vi "Initialize MeasurementLink Session.vi"(7 "remote connection options":T2, 8 "error in":errorcluster, 9 "initialize and close session behavior":T1, 10 "session initialization parameters":T3, 11 "session factory in":refnum<class "Keysight_34401A-DMM.lvclass">) -> (0 "error out":errorcluster, 2 "session out":variant, 3 "session factory out":refnum<class "Keysight_34401A-DMM.lvclass">)   [LabVIEW 2020, in "Keysight_34401A-DMM.lvclass"]
doc: "Creates a new session using the provided <b>session initialization parameters</b>. If the session represents a remote session, <b>initialize and close session behavior</b> determines whether creating the local session creates a new session on the server or attaches to an existing session on the server."
uses:
  Keysight_34401A-DMM.lvclass
  <vilib>/MeasurementLink/MeasurementLink Instrument/ISession Factory/Session Initialization Parameters.ctl
  <vilib>/MeasurementLink/MeasurementLink Instrument/ISession Factory/Remote Connection Options.ctl
  <vilib>/MeasurementLink/MeasurementLink Instrument/ISession Factory/Initialize and Close Session Behavior.ctl
  Keysight_34401A-DMM.lvclass/Keysight_34401A-DMM.ctl
  <vilib>/MeasurementLink/MeasurementLink Instrument/ISession Factory/ISession Factory.lvclass
  <instrlib>/Agilent 34401/Public/Initialize.vi
  <instrlib>/Agilent 34401/Agilent 34401.lvlib
  SubVI/Get VISA gRPC Open Close Behavior.vi
  <vilib>/NI-VISA/VISA Open for gRPC Session.vi
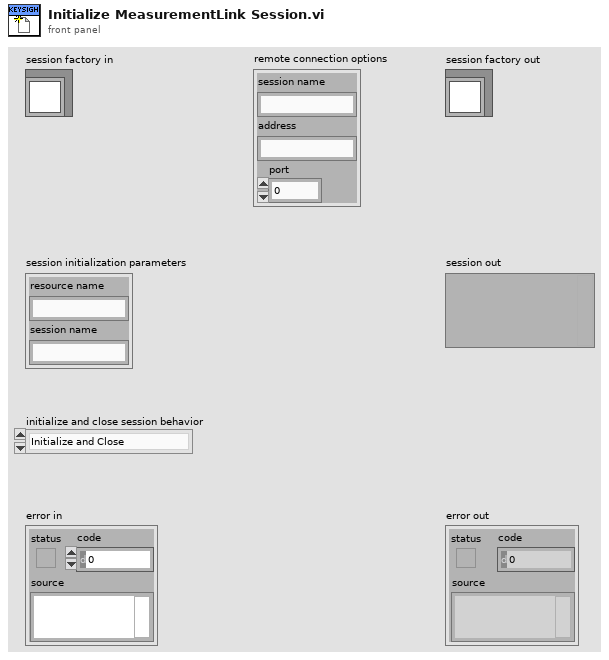
[diagram p1: front panel]
types:
  T1 = typedef "MeasurementLink Instrument.lvlib/ISession Factory.lvclass/Initialize and Close Session Behavior.ctl" = enum16{"Initialize and Close", "Attach and Detach", "Initialize and Detach", "Attach and Close"}
  T2 = typedef "MeasurementLink Instrument.lvlib/ISession Factory.lvclass/Remote Connection Options.ctl" = cluster{"session name":string, "address":string, "port":u32}
  T3 = typedef "MeasurementLink Instrument.lvlib/ISession Factory.lvclass/Session Initialization Parameters.ctl" = cluster{"resource name":string, "session name":string}
  T4 = typedef "VISA gRPC Open Close Behavior.ctl" = enum16{"Auto", "Initialize and Close", "Attach and Detach", "Initialize and Detach", "Attach and Close"}
  T5 = cluster{"Baud Rate":u32, "Parity":u16, "Data Bits":u16}
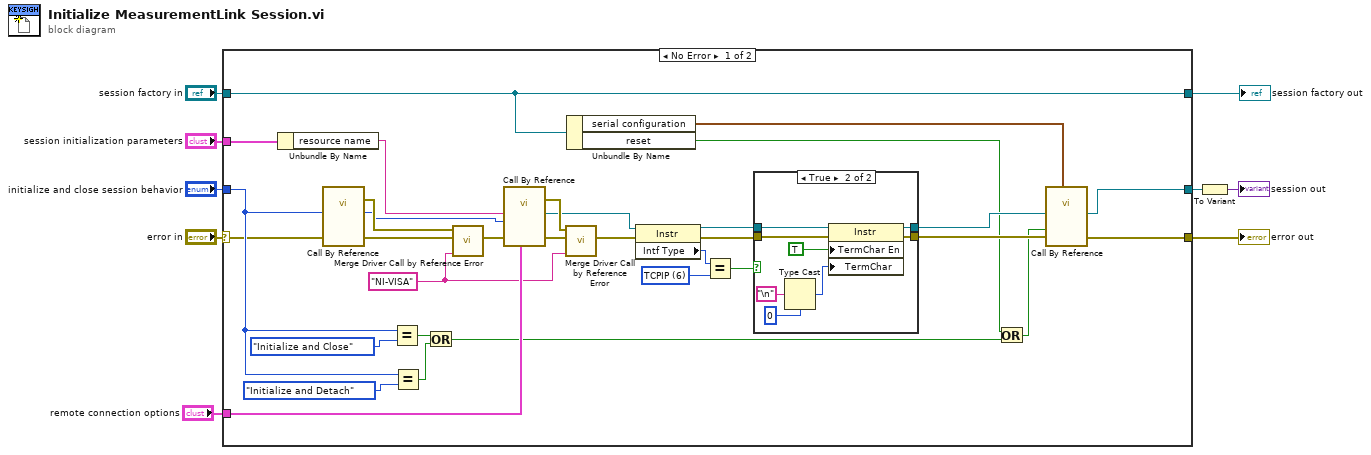
[diagram p0: block diagram]
diagram:
  n1 = case shown="No Error" "error in" {
    selector: "error in" -> [w36 w52]
    tunnel: [w10 w52] -> w9
    tunnel: "session factory in" -> [w15 w53]
    tunnel: "initialize and close session behavior" -> [w37 _]
    tunnel: "remote connection options" -> [w32 _]
    tunnel: [w15 w53] -> w4
    tunnel: [w31 _] -> w3
    tunnel: "session initialization parameters" -> [w30 _]
    frame No Error {
      w23 = u16 6 items=["GPIB"=1, "VXI"=2, "GPIB-VXI"=3, "Serial"=4, "PXI"=5, "TCPIP"=6, "USB"=7, "FireWire"=9] ("Interface Information:Interface Type")
      w26 = "NI-VISA" ("driver name")
      n2 = Unbundle By Name(w30) -> ("resource name"=w29:string)
      n3 = call-by-ref "?"("initialize session behavior"=w37, "error in (no error)"=w36) -> (error out=w34:errorcluster, "open/close behavior"=w16:T4, 15:"error out"=w35:errorcluster)  [unwired: 14 in, 1 out]
      n4 = Equal?(x=w37, y=Initialize_and_Close_Session_Behavior."Initialize and Close" ("initialize session behavior")) -> (x = y?=w39:bool)
      n5 = Equal?(x=w37, y=Initialize_and_Close_Session_Behavior."Initialize and Detach" ("initialize session behavior")) -> (x = y?=w38:bool)
      n6 = Or(x=w39, y=w38) -> (x .or. y?=w13:bool)
      n7 = call <vilib>:"Merge Driver Call by Reference Error.vi"("driver name"=w26, "called vi error"=w35, "call by ref error"=w34) -> ("error out"=w33:errorcluster)  [unwired: 8 in]
      n8 = call-by-ref "?"("gRPC Options"=w32, "error in (no error)"=w33, "Open/Close Behavior"=w16, "VISA resource name"=w29) -> (error out=w27:errorcluster, 0:"error out"=w28:errorcluster, "VISA resource name out"=w18:refnum<visa-resource-name>)  [unwired: 8 in, 1 out]
      n9 = call <vilib>:"Merge Driver Call by Reference Error.vi"("driver name"=w26, "called vi error"=w28, "call by ref error"=w27) -> ("error out"=w21:errorcluster)  [unwired: 8 in]
      n10 = Unbundle By Name(w15) -> ("serial configuration"=w14:T5, "reset"=w11:bool)
      n11 = property class="Instr"(reference=w18, error in=w21) -> (reference out=w19:refnum<visa-resource-name>, error out=w20:errorcluster, "Intf Type"=w22:u16)
      n12 = Equal?(x=w22, y=w23) -> (x = y?=w17:bool)
      n13 = case shown="True" w17 {
        tunnel: w20 -> [w43 w51]
        tunnel: [w43 w50] -> w25
        tunnel: w19 -> [w42 w49]
        tunnel: [w42 w48] -> w24
        frame False {
        }
        frame True {
          n14 = Type Cast(type=u8 0, x="\n" ("Line Feed Constant")) -> (*(type *) &x=w44:u8)
          n15 = property class="Instr"(reference=w49, error in=w51, "TermChar En"=TRUE ("Message Based Settings:Termination Character Enable"), "TermChar"=w44) -> (reference out=w48:refnum<visa-resource-name>, error out=w50:errorcluster)
        }
      }
      n16 = Or(x=w11, y=w13) -> (x .or. y?=w12:bool)
      n17 = call-by-ref "?"("Serial Configuration"=w14, "error in (no error)"=w25, "Reset (True)"=w12, "VISA resource name"=w24) -> ("error out"=w10:errorcluster, "VISA resource name out"=w31:refnum<visa-resource-name>)  [unwired: 8 in, 2 out]
    }
    frame Error {
    }
  }
  "error out" <- w9
  "session factory out" <- w4
  n18 = To Variant(anything=w3) -> (Variant=→"session out":variant)
